vi "Plot Waypoint Tangent.vi"() -> ()   [LabVIEW 2019]
panel:
  out "T_i":cluster{dbl, dbl}
  in  "point c":cluster{"x":dbl, "y":dbl}
  in  "point b":cluster{"x":dbl, "y":dbl}
  in  "point a":cluster{"x":dbl, "y":dbl}
  out "XY Graph":cluster{"X":dbl, "Y":dbl}[](graph)
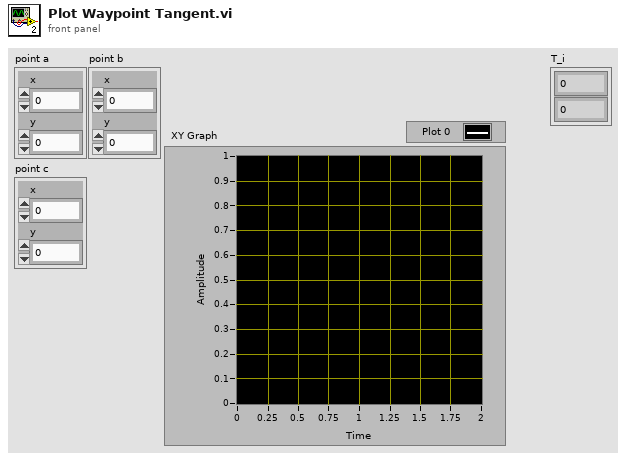
[diagram p1: front panel]
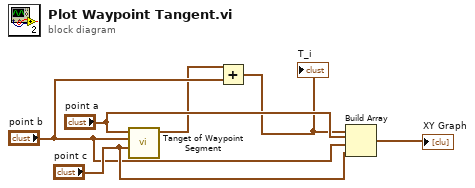
[diagram p0: block diagram]
diagram:
  n1 = call "Tanget of Waypoint Segment.vi"("point c"="point c", "point b"="point b", "point a"="point a") -> ("T_i"=w1:cluster{dbl, dbl})  [unwired: 8 in]
  n2 = Add(x=w1, y="point b") -> (x+y=w3:cluster{dbl, dbl})
  "T_i" <- w3
  n3 = Build Array(w3, "point a", "point b", "point c") -> (→"XY Graph":cluster{"x":dbl, "y":dbl}[])
